vi "ExSubCreateR3FileDisplay.vi"(2 "error in (no error)":errorcluster, 3 "File and Display Name":string, 5 "Camera Handle":u32) -> (0 "error out":errorcluster, 1 "Handles Out":T1)   [LabVIEW 2010]
panel:
  # "ExSubCreateFileDisplay:\nThis is a SubVI that creates a file, display \nand image objects and returns the handles \nbundled in a cluster that includes a pulser \nand camera handle"
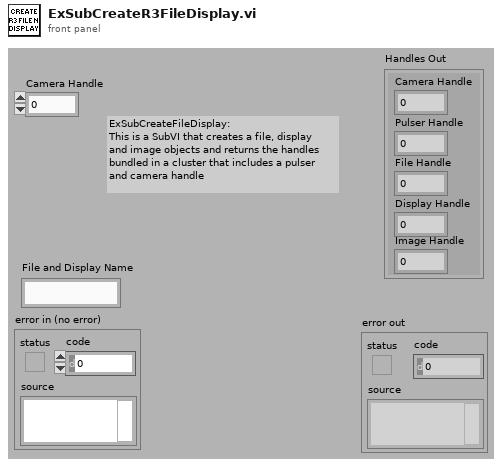
[diagram p1: front panel]
types:
  T1 = cluster{"Camera Handle":u32, "Pulser Handle":u32, "File Handle":u32, "Display Handle":u32, "Image Handle":u32}
  T2 = cluster{"Camera Handle":u32, i32, "File Handle":u32, "Display Handle":u32, "Image Handle":u32}
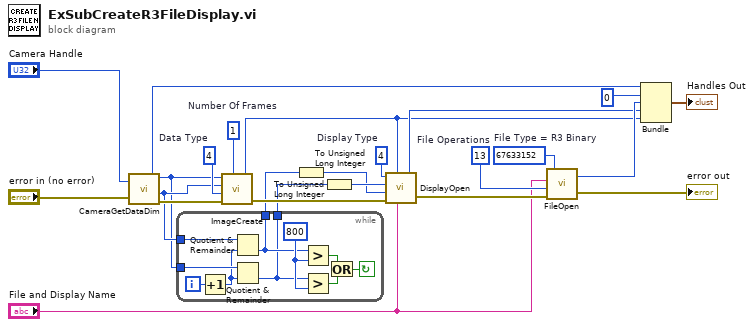
[diagram p0: block diagram]
diagram:
  w8 = u32 1  # Number Of Frames
  w9 = u32 4  # Display Type
  w10 = u32 4  # Data Type
  w12 = 13  # File Operations
  w13 = 67633152  # File Type = R3 Binary
  n1 = call <userlib>:"CameraGetDataDim.vi"("Camera Handle"="Camera Handle", "error in"="error in (no error)") -> ("Camera Handle"=w18:u32, "Xdim"=w2:u32, "Ydim"=w3:u32, "error out"=w24:errorcluster)
  n2 = while {
    tunnel: w3 -> [w33]
    tunnel: w2 -> [w32]
    tunnel: [w27] -> w7
    tunnel: [w26] -> w6
    i -> [w31]
    stop <- w28 continue-if-true
    w34 = 800
    n3 = Increment(x=w31) -> (x+1=w25:i32)
    n4 = Quotient & Remainder(x=w33, y=w25) -> (floor(x/y)=w27:u32)  [unwired: 1 out]
    n5 = Quotient & Remainder(x=w32, y=w25) -> (floor(x/y)=w26:u32)  [unwired: 1 out]
    n6 = Greater?(x=w27, y=w34) -> (0:w30:bool)
    n7 = Greater?(x=w26, y=w34) -> (0:w29:bool)
    n8 = Or(x=w30, y=w29) -> (x .or. y?=w28:bool)
  }
  n9 = call <userlib>:"ImageCreate.vi"("X dimension"=w2, "Y dimension"=w3, "Data Type"=w10, "error in"=w24, "Number Of Frames"=w8) -> ("Image Handle"=w15:u32, "error out"=w23:errorcluster)
  n10 = To Unsigned Long Integer(number=w7) -> (unsigned 32bit integer=w4:u32)
  n11 = To Unsigned Long Integer(number=w6) -> (unsigned 32bit integer=w5:u32)
  n12 = call <userlib>:"DisplayOpen.vi"("Display Title"="File and Display Name", "Image Handle"=w15, "error in"=w23, "Display Height"=w4, "Display Width"=w5, "Display Type"=w9) -> ("error out"=w22:errorcluster, "Display Handle"=w16:u32)
  n13 = call <userlib>:"FileOpen.vi"("error in"=w22, "File Operations"=w12, "FileName"="File and Display Name", "File Type"=w13) -> ("error out"=→"error out":errorcluster, "File Handle"=w17:u32)
  n14 = Bundle("Camera Handle"=w18, 0, "File Handle"=w17, "Display Handle"=w16, "Image Handle"=w15) -> (→"Handles Out":T2)  [unwired: 1 in]
